vi "auto Scan  Relay Board ID.vi"(8 "error in (no error)":errorcluster) -> (0 "error out":errorcluster, 2 "RelayBoard Infor":T1={"VISA resource name"="", "Board Address"=0, "baudrate(9600)"=3} {"baudrate(9600)" items=["4800"=2, "9600"=3, "19200"=4]})   [LabVIEW 2016]
uses:
  type defs/Relay Board Infor.ctl
  type defs/baudrate.ctl
  <vilib>/Instr/_visa.llb/VISA Configure Serial Port (Instr).vi
  MB _relays.lvlib
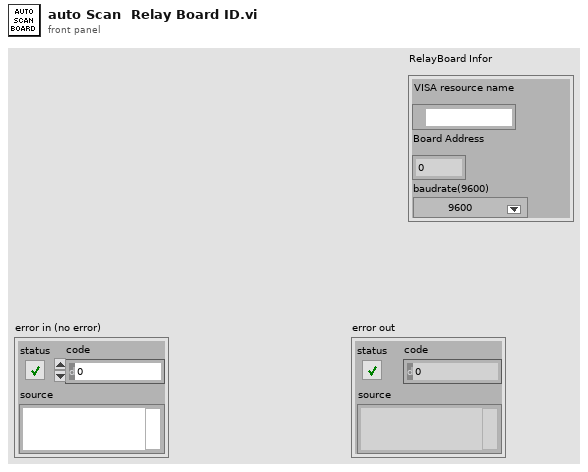
[diagram p1: front panel]
types:
  T1 = typedef "Relay Board Infor.ctl" = cluster{"VISA resource name":refnum<visa-resource-name>, "Board Address":u8, "baudrate(9600)":T2}
  T2 = typedef "MB _relays.lvlib/baudrate.ctl" = u8
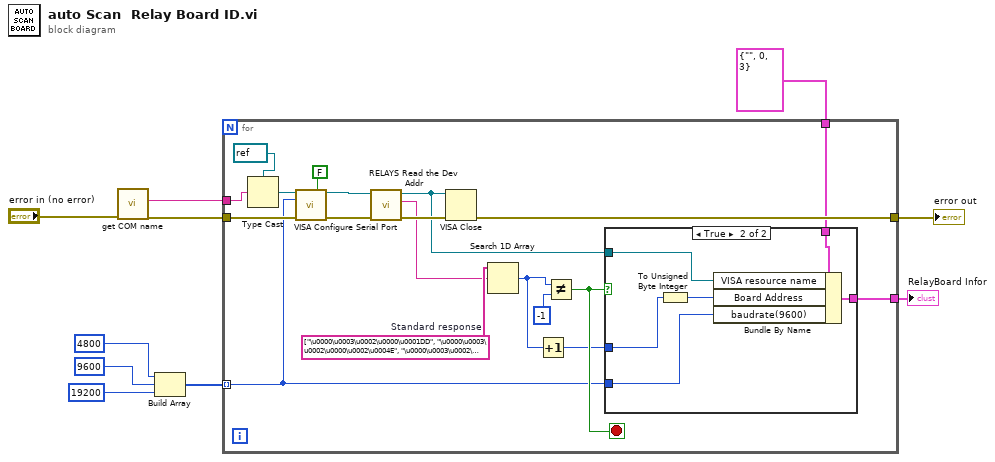
[diagram p0: block diagram]
diagram:
  n1 = call "get COM name.vi"("error in (no error)"="error in (no error)") -> ("error out"=w8:errorcluster, "COMport Name"=w9:string)  [unwired: 9 in]
  n2 = Build Array(u32 4800 ("baud rate (9600)"), u32 9600 ("baud rate (9600)"), u32 19200 ("baud rate (9600)")) -> (w6:u32[])
  n3 = for {
    tunnel: w9 -> [w29]
    tunnel: w8 -> [w26]
    tunnel: w6 -> [w14] mode=indexing
    tunnel: [w20] -> w5
    tunnel: T1 {"VISA resource name"="", "Board Address"=0, "baudrate(9600)"=3} ("RelayBoard Infor") -> [w16]
    tunnel: [w13] -> w1
    stop <- w17 stop-if-true
    w21 = string[] ["\u0000\u0003\u0002\u0000\u0001DD", "\u0000\u0003\u0002\u0000\u0002\u0004E", "\u0000\u0003\u0002\u0000\u0003Ņ", "\u0000\u0003\u0002\u0000\u0004„G", "\u0000\u0003\u0002\u0000\u0005E‡", "\u0000\u0003\u0002\u0000\u0006\u0005†", "\u0000\u0003\u0002\u0000\u0007ÄF", "\u0000\u0003\u0002\u0000\b„B", "\u0000\u0003\u0002\u0000\tE‚", "\u0000\u0003\u0002\u0000\n\u0005ƒ", "\u0000\u0003\u0002\u0000\u000bÄC", "\u0000\u0003\u0002\u0000\f", "\u0000\u0003\u0002\u0000\rDA", "\u0000\u0003\u0002\u0000\u000e\u0004@", "\u0000\u0003\u0002\u0000\u000fŀ", "\u0000\u0003\u0002\u0000\u0010„H", "\u0000\u0003\u0002\u0000\u0011Eˆ", "\u0000\u0003\u0002\u0000\u0012\u0005‰", "\u0000\u0003\u0002\u0000\u0013ÄI", "\u0000\u0003\u0002\u0000\u0014…‹", "\u0000\u0003\u0002\u0000\u0015DK", "\u0000\u0003\u0002\u0000\u0016\u0004J", "\u0000\u0003\u0002\u0000\u0017Ŋ", "\u0000\u0003\u0002\u0000\u0018…Ž", "\u0000\u0003\u0002\u0000\u0019DN", "\u0000\u0003\u0002\u0000\u001a\u0004O", "\u0000\u0003\u0002\u0000\u001bŏ", "\u0000\u0003\u0002\u0000\u001c„M", "\u0000\u0003\u0002\u0000\u001dE", "\u0000\u0003\u0002\u0000\u001e\u0005Œ", "\u0000\u0003\u0002\u0000\u001fÄL", "\u0000\u0003\u0002\u0000 „\\", "\u0000\u0003\u0002\u0000!Eœ", "\u0000\u0003\u0002\u0000\"\u0005", "\u0000\u0003\u0002\u0000#Ä]", "\u0000\u0003\u0002\u0000$…Ÿ", "\u0000\u0003\u0002\u0000%D_", "\u0000\u0003\u0002\u0000&\u0004^", "\u0000\u0003\u0002\u0000'Ş", "\u0000\u0003\u0002\u0000(…š", "\u0000\u0003\u0002\u0000)DZ", "\u0000\u0003\u0002\u0000*\u0004[", "\u0000\u0003\u0002\u0000+ś", "\u0000\u0003\u0002\u0000,„Y", "\u0000\u0003\u0002\u0000-E™", "\u0000\u0003\u0002\u0000.\u0005˜", "\u0000\u0003\u0002\u0000/ÄX", "\u0000\u0003\u0002\u00000", "\u0000\u0003\u0002\u00001DP", "\u0000\u0003\u0002\u00002\u0004Q", "\u0000\u0003\u0002\u00003ő", "\u0000\u0003\u0002\u00004„S", "\u0000\u0003\u0002\u00005E“", "\u0000\u0003\u0002\u00006\u0005’", "\u0000\u0003\u0002\u00007ÄR", "\u0000\u0003\u0002\u00008„V", "\u0000\u0003\u0002\u00009E–", "\u0000\u0003\u0002\u0000:\u0005—", "\u0000\u0003\u0002\u0000;ÄW", "\u0000\u0003\u0002\u0000<…•", "\u0000\u0003\u0002\u0000=DU", "\u0000\u0003\u0002\u0000>\u0004T", "\u0000\u0003\u0002\u0000?Ŕ", "\u0000\u0003\u0002\u0000@„t", "\u0000\u0003\u0002\u0000AE´", "\u0000\u0003\u0002\u0000B\u0005µ", "\u0000\u0003\u0002\u0000CÄu", "\u0000\u0003\u0002\u0000D…·", "\u0000\u0003\u0002\u0000EDw", "\u0000\u0003\u0002\u0000F\u0004v", "\u0000\u0003\u0002\u0000GŶ", "\u0000\u0003\u0002\u0000H…²", "\u0000\u0003\u0002\u0000IDr", "\u0000\u0003\u0002\u0000J\u0004s", "\u0000\u0003\u0002\u0000Kų", "\u0000\u0003\u0002\u0000L„q", "\u0000\u0003\u0002\u0000ME±", "\u0000\u0003\u0002\u0000N\u0005°", "\u0000\u0003\u0002\u0000OÄp", "\u0000\u0003\u0002\u0000P…¸", "\u0000\u0003\u0002\u0000QDx", "\u0000\u0003\u0002\u0000R\u0004y", "\u0000\u0003\u0002\u0000SŹ", "\u0000\u0003\u0002\u0000T„{", "\u0000\u0003\u0002\u0000UE»", "\u0000\u0003\u0002\u0000V\u0005º", "\u0000\u0003\u0002\u0000WÄz", "\u0000\u0003\u0002\u0000X„~", "\u0000\u0003\u0002\u0000YE¾", "\u0000\u0003\u0002\u0000Z\u0005¿", "\u0000\u0003\u0002\u0000[Ä", "\u0000\u0003\u0002\u0000\\…½", "\u0000\u0003\u0002\u0000]D}", "\u0000\u0003\u0002\u0000^\u0004|", "\u0000\u0003\u0002\u0000_ż", "\u0000\u0003\u0002\u0000`…¬", "\u0000\u0003\u0002\u0000aDl", "\u0000\u0003\u0002\u0000b\u0004m", "\u0000\u0003\u0002\u0000cŭ", "\u0000\u0003\u0002\u0000d„o", "\u0000\u0003\u0002\u0000eE¯", "\u0000\u0003\u0002\u0000f\u0005®", "\u0000\u0003\u0002\u0000gÄn", "\u0000\u0003\u0002\u0000h„j", "\u0000\u0003\u0002\u0000iEª", "\u0000\u0003\u0002\u0000j\u0005«", "\u0000\u0003\u0002\u0000kÄk", "\u0000\u0003\u0002\u0000l…©", "\u0000\u0003\u0002\u0000mDi", "\u0000\u0003\u0002\u0000n\u0004h", "\u0000\u0003\u0002\u0000oŨ", "\u0000\u0003\u0002\u0000p„`", "\u0000\u0003\u0002\u0000qE ", "\u0000\u0003\u0002\u0000r\u0005¡", "\u0000\u0003\u0002\u0000sÄa", "\u0000\u0003\u0002\u0000t…£", "\u0000\u0003\u0002\u0000uDc", "\u0000\u0003\u0002\u0000v\u0004b", "\u0000\u0003\u0002\u0000wŢ", "\u0000\u0003\u0002\u0000x…¦", "\u0000\u0003\u0002\u0000yDf", "\u0000\u0003\u0002\u0000z\u0004g", "\u0000\u0003\u0002\u0000{ŧ", "\u0000\u0003\u0002\u0000|„e", "\u0000\u0003\u0002\u0000}E¥", "\u0000\u0003\u0002\u0000~\u0005¤", "\u0000\u0003\u0002\u0000Äd", "\u0000\u0003\u0002\u0000€„$", "\u0000\u0003\u0002\u0000Eä", "\u0000\u0003\u0002\u0000‚\u0005å", "\u0000\u0003\u0002\u0000ƒÄ%", "\u0000\u0003\u0002\u0000„…ç", "\u0000\u0003\u0002\u0000…D'", "\u0000\u0003\u0002\u0000†\u0004&", "\u0000\u0003\u0002\u0000‡Åæ", "\u0000\u0003\u0002\u0000ˆ…â", "\u0000\u0003\u0002\u0000‰D\"", "\u0000\u0003\u0002\u0000Š\u0004#", "\u0000\u0003\u0002\u0000‹Åã", "\u0000\u0003\u0002\u0000Œ„!", "\u0000\u0003\u0002\u0000Eá", "\u0000\u0003\u0002\u0000Ž\u0005à", "\u0000\u0003\u0002\u0000Ä ", "\u0000\u0003\u0002\u0000è", "\u0000\u0003\u0002\u0000‘D(", "\u0000\u0003\u0002\u0000’\u0004)", "\u0000\u0003\u0002\u0000“Åé", "\u0000\u0003\u0002\u0000”„+", "\u0000\u0003\u0002\u0000•Eë", "\u0000\u0003\u0002\u0000–\u0005ê", "\u0000\u0003\u0002\u0000—Ä*", "\u0000\u0003\u0002\u0000˜„.", "\u0000\u0003\u0002\u0000™Eî", "\u0000\u0003\u0002\u0000š\u0005ï", "\u0000\u0003\u0002\u0000›Ä/", "\u0000\u0003\u0002\u0000œ…í", "\u0000\u0003\u0002\u0000D-", "\u0000\u0003\u0002\u0000ž\u0004,", "\u0000\u0003\u0002\u0000ŸÅì", "\u0000\u0003\u0002\u0000 …ü", "\u0000\u0003\u0002\u0000¡D<", "\u0000\u0003\u0002\u0000¢\u0004=", "\u0000\u0003\u0002\u0000£Åý", "\u0000\u0003\u0002\u0000¤„?", "\u0000\u0003\u0002\u0000¥Eÿ", "\u0000\u0003\u0002\u0000¦\u0005þ", "\u0000\u0003\u0002\u0000§Ä>", "\u0000\u0003\u0002\u0000▌:", "\u0000\u0003\u0002\u0000©Eú", "\u0000\u0003\u0002\u0000ª\u0005û", "\u0000\u0003\u0002\u0000«Ä;", "\u0000\u0003\u0002\u0000¬…ù", "\u0000\u0003\u0002\u0000­D9", "\u0000\u0003\u0002\u0000®\u00048", "\u0000\u0003\u0002\u0000¯Åø", "\u0000\u0003\u0002\u0000皠0", "\u0000\u0003\u0002\u0000±Eð", "\u0000\u0003\u0002\u0000²\u0005ñ", "\u0000\u0003\u0002\u0000衬1", "\u0000\u0003\u0002\u0000´…ó", "\u0000\u0003\u0002\u0000µD3", "\u0000\u0003\u0002\u0000¶\u00042", "\u0000\u0003\u0002\u0000·Åò", "\u0000\u0003\u0002\u0000¸…ö", "\u0000\u0003\u0002\u0000¹D6", "\u0000\u0003\u0002\u0000º\u00047", "\u0000\u0003\u0002\u0000»Å÷", "\u0000\u0003\u0002\u0000紕5", "\u0000\u0003\u0002\u0000½Eõ", "\u0000\u0003\u0002\u0000¾\u0005ô", "\u0000\u0003\u0002\u0000磕4", "\u0000\u0003\u0002\u0000À…Ô", "\u0000\u0003\u0002\u0000ÁD\u0014", "\u0000\u0003\u0002\u0000Â\u0004\u0015", "\u0000\u0003\u0002\u0000ÃÅÕ", "\u0000\u0003\u0002\u0000Ą\u0017", "\u0000\u0003\u0002\u0000ÅE×", "\u0000\u0003\u0002\u0000Æ\u0005Ö", "\u0000\u0003\u0002\u0000悄\u0016", "\u0000\u0003\u0002\u0000Ȅ\u0012", "\u0000\u0003\u0002\u0000ÉEÒ", "\u0000\u0003\u0002\u0000Ê\u0005Ó", "\u0000\u0003\u0002\u0000四\u0013", "\u0000\u0003\u0002\u0000Ì…Ñ", "\u0000\u0003\u0002\u0000ÍD\u0011", "\u0000\u0003\u0002\u0000Î\u0004\u0010", "\u0000\u0003\u0002\u0000ÏÅÐ", "\u0000\u0003\u0002\u0000Є\u0018", "\u0000\u0003\u0002\u0000ÑEØ", "\u0000\u0003\u0002\u0000Ò\u0005Ù", "\u0000\u0003\u0002\u0000幽\u0019", "\u0000\u0003\u0002\u0000Ô…Û", "\u0000\u0003\u0002\u0000ÕD\u001b", "\u0000\u0003\u0002\u0000Ö\u0004\u001a", "\u0000\u0003\u0002\u0000×ÅÚ", "\u0000\u0003\u0002\u0000Ø…Þ", "\u0000\u0003\u0002\u0000ÙD\u001e", "\u0000\u0003\u0002\u0000Ú\u0004\u001f", "\u0000\u0003\u0002\u0000ÛÅß", "\u0000\u0003\u0002\u0000܄\u001d", "\u0000\u0003\u0002\u0000ÝEÝ", "\u0000\u0003\u0002\u0000Þ\u0005Ü", "\u0000\u0003\u0002\u0000ßÄ\u001c", "\u0000\u0003\u0002\u0000à„\f", "\u0000\u0003\u0002\u0000áEÌ", "\u0000\u0003\u0002\u0000â\u0005Í", "\u0000\u0003\u0002\u0000ãÄ\r", "\u0000\u0003\u0002\u0000ä…Ï", "\u0000\u0003\u0002\u0000åD\u000f", "\u0000\u0003\u0002\u0000æ\u0004\u000e", "\u0000\u0003\u0002\u0000çÅÎ", "\u0000\u0003\u0002\u0000è…Ê", "\u0000\u0003\u0002\u0000éD\n", "\u0000\u0003\u0002\u0000ê\u0004\u000b", "\u0000\u0003\u0002\u0000ëÅË", "\u0000\u0003\u0002\u0000ì„\t", "\u0000\u0003\u0002\u0000íEÉ", "\u0000\u0003\u0002\u0000î\u0005È", "\u0000\u0003\u0002\u0000ïÄ\b", "\u0000\u0003\u0002\u0000ð…À", "\u0000\u0003\u0002\u0000ñD\u0000", "\u0000\u0003\u0002\u0000ò\u0004\u0001", "\u0000\u0003\u0002\u0000óÅÁ", "\u0000\u0003\u0002\u0000ô„\u0003", "\u0000\u0003\u0002\u0000õEÃ", "\u0000\u0003\u0002\u0000ö\u0005Â", "\u0000\u0003\u0002\u0000÷Ä\u0002", "\u0000\u0003\u0002\u0000ø„\u0006", "\u0000\u0003\u0002\u0000ùEÆ", "\u0000\u0003\u0002\u0000ú\u0005Ç", "\u0000\u0003\u0002\u0000ûÄ\u0007", "\u0000\u0003\u0002\u0000ü…Å", "\u0000\u0003\u0002\u0000ýD\u0005", "\u0000\u0003\u0002\u0000þ\u0004\u0004", "\u0000\u0003\u0002\u0000ÿÅÄ"]  # Standard response
    n4 = Type Cast(type=refnum<visa-resource-name> refnum ("VISA resource name"), x=w29) -> (*(type *) &x=w28:refnum<visa-resource-name>)
    n5 = call-poly "VISA Configure Serial Port"("VISA resource name"=w28, "Enable Termination\nChar (T)"=FALSE ("Enable Termination\nChar (T)"), "baud rate (9600)"=w14, "error in (no error)"=w26) -> ("VISA resource name out"=w25:refnum<visa-resource-name>, "error out"=w24:errorcluster)  [unwired: 10 in]
    n6 = call "RELAYS Read the Dev Addr.vi"("error in (no error)"=w24, "VISA resource name"=w25) -> ("error out"=w23:errorcluster, "ack"=w12:string, "VISA resource name out"=w11:refnum<visa-resource-name>)  [unwired: 7 in]
    n7 = VISA Close(VISA resource name=w11, error in (no error)=w23) -> (error out=w20:errorcluster)
    n8 = Search 1D Array(1D array=w21, element=w12) -> (index of element=w18:i32)  [unwired: 1 in]
    n9 = Increment(x=w18) -> (x+1=w15:i32)
    n10 = Not Equal?(x=w18, y=-1) -> (x != y?=w17:bool)
    n11 = case shown="True" w17 {
      tunnel: w16 -> [w30 w36]
      tunnel: w15 -> [_ w32]
      tunnel: w14 -> [_ w33]
      tunnel: [w30 w35] -> w13
      tunnel: w11 -> [_ w34]
      frame False {
      }
      frame True {
        n12 = To Unsigned Byte Integer(number=w32) -> (unsigned 8bit integer=w31:u8)
        n13 = Bundle By Name(cluster=w36, "VISA resource name"=w34, "Board Address"=w31, "baudrate(9600)"=w33) -> (w35:T1)
      }
    }
  }
  "error out" <- w5
  "RelayBoard Infor" <- w1
